vi "Prepare XCP address (SubVI).vi"(11 "XCP file Address":string) -> (3 "Polarity Address":u32[](array[numeric]) format="%.0x")   [LabVIEW 2025]
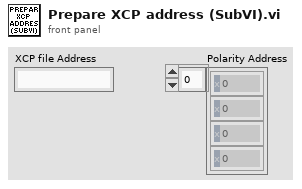
[diagram p1: front panel]
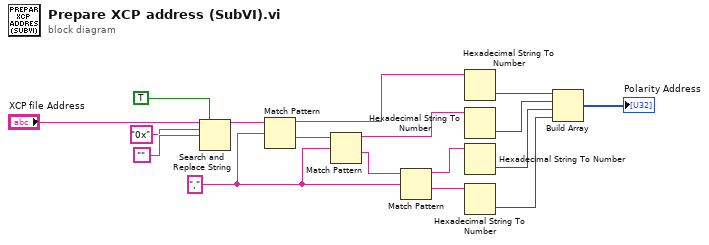
[diagram p0: block diagram]
diagram:
  w12 = "," ("regular expression")
  n1 = Search and Replace String(replace all?=TRUE ("replace all? (F)"), input string="XCP file Address", search string="0x", replace string="") -> (result string=w13:string)  [unwired: 4 in, 3 out]
  n2 = Match Pattern(string=w13, regular expression=w12) -> (before substring=w8:string, after substring=w10:string)  [unwired: 1 in, 2 out]
  n3 = Match Pattern(string=w10, regular expression=w12) -> (before substring=w7:string, after substring=w11:string)  [unwired: 1 in, 2 out]
  n4 = Match Pattern(string=w11, regular expression=w12) -> (before substring=w6:string, after substring=w17:string)  [unwired: 1 in, 2 out]
  n5 = Hexadecimal String To Number(string=w8) -> (number=w5:u32)  [unwired: 2 in, 1 out]
  n6 = Hexadecimal String To Number(string=w7) -> (number=w4:u32)  [unwired: 2 in, 1 out]
  n7 = Hexadecimal String To Number(string=w6) -> (number=w3:u32)  [unwired: 2 in, 1 out]
  n8 = Hexadecimal String To Number(string=w17) -> (number=w2:u32)  [unwired: 2 in, 1 out]
  n9 = Build Array(w5, w4, w3, w2) -> (→"Polarity Address":u32[])
